vi "MongoDB.SimpleExample.vi"() -> ()   [LabVIEW 2014]
uses:
  MongoDB.Collection.lvclass
  MongoDB.Database.lvclass
  MongoDB.Client.lvclass
panel:
  out "Result 2":string
  out "Result":string
  out "Array 2":string[](array[string])
  out "Results":string[](array[string])
  out "Array":string[](array[string])
  in  "collectionName":string
  in  "databaseName":string
  in  "connectionString":string
  out "CollectionNames":string[](array[string])
  out "UserNames":string[](array[string])
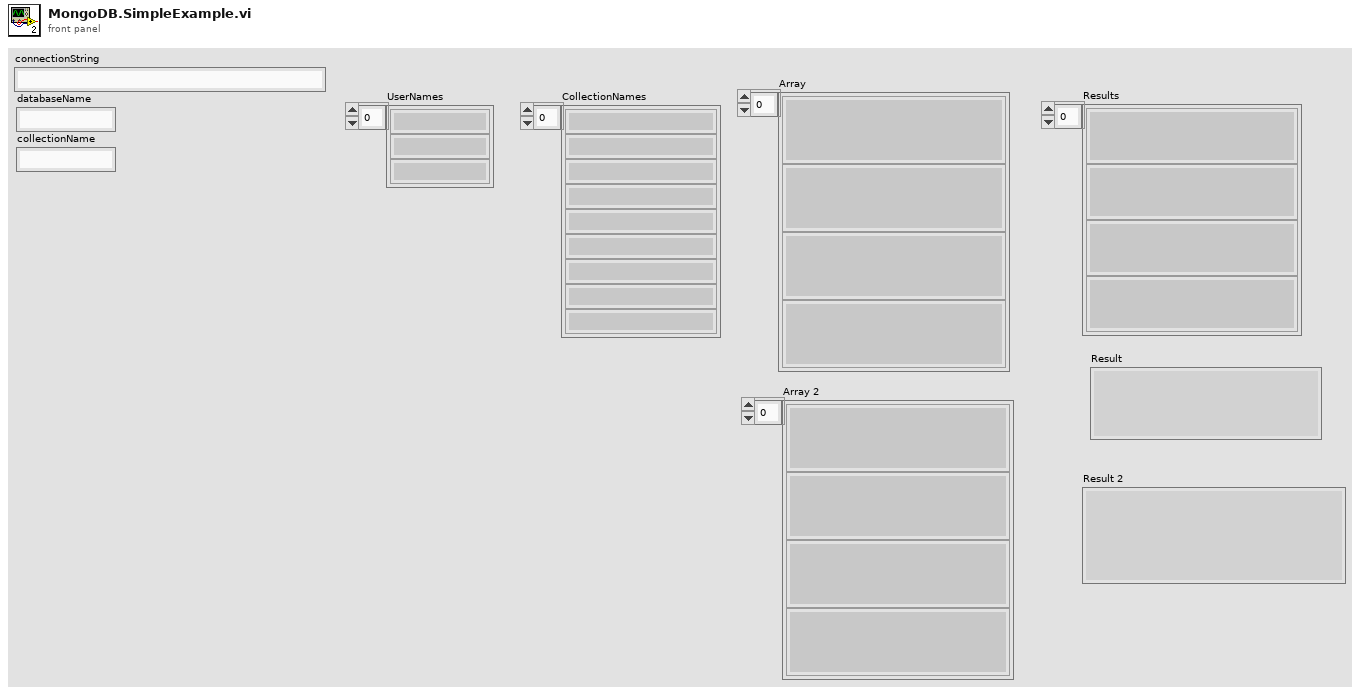
[diagram p1: front panel]
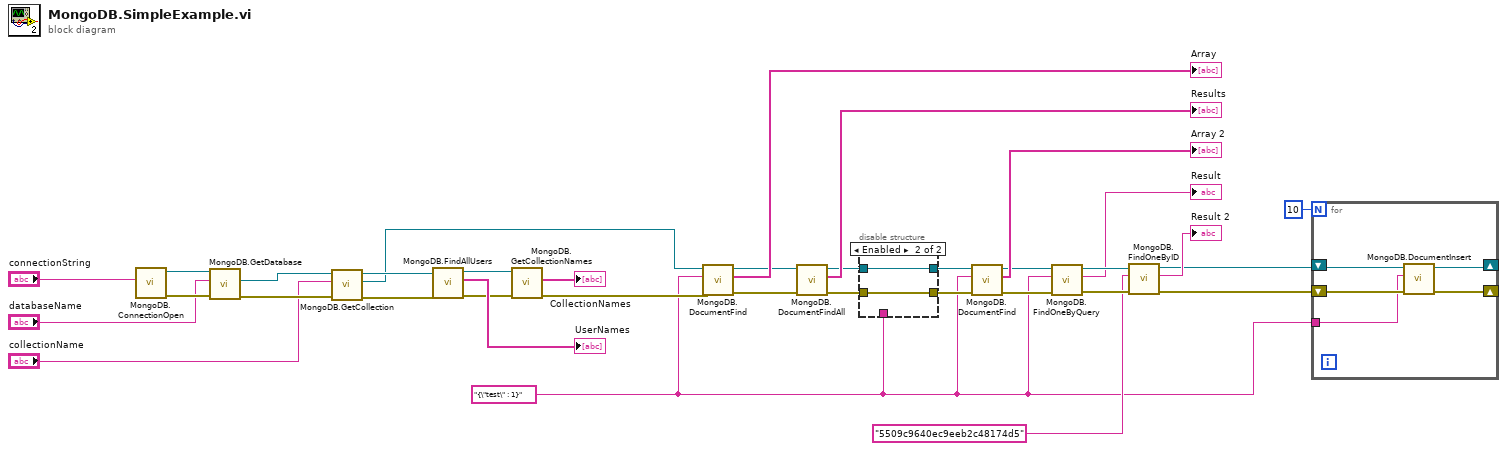
[diagram p0: block diagram]
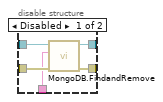
[diagram p2: hidden frame]
diagram:
  w1 = "{\"test\" : 1}" ("value")
  n1 = call "MongoDB.ConnectionOpen.vi"("connectionString"="connectionString") -> ("error out"=w34:errorcluster, "MongoDB out"=w35:refnum<class "MongoDB.Client.lvclass">)  [unwired: 9 in]
  n2 = call "MongoDB.GetDatabase.vi"("error in (no error)"=w34, "databaseName"="databaseName", "MongoDB.Connection in"=w35) -> ("error out"=w32:errorcluster, "MongoDB.Database out"=w33:refnum<class "MongoDB.Database.lvclass">)  [unwired: 6 in, 1 out]
  n3 = call "MongoDB.GetCollection.vi"("error in (no error)"=w32, "collectionName"="collectionName", "MongoDB.Database in"=w33) -> ("error out"=w27:errorcluster, "MongoDB.Collection out"=w22:refnum<class "MongoDB.Collection.lvclass">, "MongoDB.Database out"=w29:refnum<class "MongoDB.Database.lvclass">)  [unwired: 6 in]
  n4 = call-dynamic "MongoDB.FindAllUsers.vi"("error in (no error)"=w27, "MongoDB.Database in"=w29) -> ("error out"=w26:errorcluster, "UserNames"=→"UserNames":string[], "MongoDB.Database out"=w25:refnum<class "MongoDB.Database.lvclass">)  [unwired: 7 in]
  n5 = call-dynamic "MongoDB.GetCollectionNames.vi"("error in (no error)"=w26, "MongoDB.Database in"=w25) -> ("error out"=w21:errorcluster, "CollectionNames"=→"CollectionNames":string[])  [unwired: 7 in, 1 out]
  n6 = call-dynamic "MongoDB.DocumentFind.vi"("error in (no error)"=w21, "value"=w1, "MongoDB.Collection in"=w22) -> ("error out"=w18:errorcluster, "Results Array"=→"Array":string[], "MongoDB.Collection out"=w19:refnum<class "MongoDB.Collection.lvclass">)  [unwired: 6 in]
  n7 = call-dynamic "MongoDB.DocumentFindAll.vi"("error in (no error)"=w18, "MongoDB.Collection in"=w19) -> ("error out"=w13:errorcluster, "Results"=→"Results":string[], "MongoDB.Collection out"=w16:refnum<class "MongoDB.Collection.lvclass">)  [unwired: 7 in]
  n8 = disable-structure shown="Enabled" {
    disable-tunnel: w16 -> [w40 w42]
    disable-tunnel: [w39 w42] -> w15
    disable-tunnel: w13 -> [w38 w41]
    disable-tunnel: [w37 w41] -> w12
    disable-tunnel: w1 -> [w36 _]
    frame Disabled {
      n9 = call-dynamic "MongoDB.FindandRemove.vi"("error in (no error)"=w38, "Query"=w36, "MongoDB.Collection in"=w40) -> ("error out"=w37:errorcluster, "MongoDB.Collection out"=w39:refnum<class "MongoDB.Collection.lvclass">)  [unwired: 7 in]
    }
    frame Enabled {
    }
  }
  n10 = call-dynamic "MongoDB.DocumentFind.vi"("error in (no error)"=w12, "value"=w1, "MongoDB.Collection in"=w15) -> ("error out"=w10:errorcluster, "Results Array"=→"Array 2":string[], "MongoDB.Collection out"=w11:refnum<class "MongoDB.Collection.lvclass">)  [unwired: 6 in]
  n11 = call-dynamic "MongoDB.FindOneByQuery.vi"("error in (no error)"=w10, "JSON Query String"=w1, "MongoDB.Collection in"=w11) -> ("error out"=w8:errorcluster, "Result"=→"Result":string, "MongoDB.Collection out"=w9:refnum<class "MongoDB.Collection.lvclass">)  [unwired: 6 in]
  n12 = call-dynamic "MongoDB.FindOneByID.vi"("error in (no error)"=w8, "JSON Query String"="5509c9640ec9eeb2c48174d5" ("value"), "MongoDB.Collection in"=w9) -> ("error out"=w2:errorcluster, "Result"=→"Result 2":string, "MongoDB.Collection out"=w3:refnum<class "MongoDB.Collection.lvclass">)  [unwired: 6 in]
  n13 = for {
    N: 10 -> [_]
    shift-right: [w45] -> _
    shift-left: w3 -> [w47]
    shift-right: [w44] -> _
    shift-left: w2 -> [w46]
    tunnel: w1 -> [w43]
    n14 = call-dynamic "MongoDB.DocumentInsert.vi"("error in (no error)"=w46, "JSON Document"=w43, "MongoDB.Collection in"=w47) -> ("error out"=w44:errorcluster, "MongoDB.Collection out"=w45:refnum<class "MongoDB.Collection.lvclass">)  [unwired: 6 in, 1 out]
  }
